vi "NaCTA_configure.vi"() -> ()   [LabVIEW 2016]
uses:
  Instrument drivers/Arduino/ctls_and_globals/Arduino tx msg cluster.ctl
panel:
  in  "Enable USB stream":bool
  in  "n":dbl=0.5
  in  "T0 offset (deg C)":dbl
  in  "P_atmos offset (Pa)":dbl
  in  "Port":refnum<visa-resource-name>
  in  "Get / Set":u8(ring) items=["Get", "Set"]
  in  "Apply temperature corrections":bool=TRUE
  in  "B":dbl=1.0
  in  "A":dbl
  out "Read-back":string
  out "Status comment":string
  in  "Address":u8=1
  # "Use this vi to configure the NaCTA 'hot-thermistor' node\nThese settings are retained in EEPROM and recalled on power-up."
  # "PN 03/02/2017"
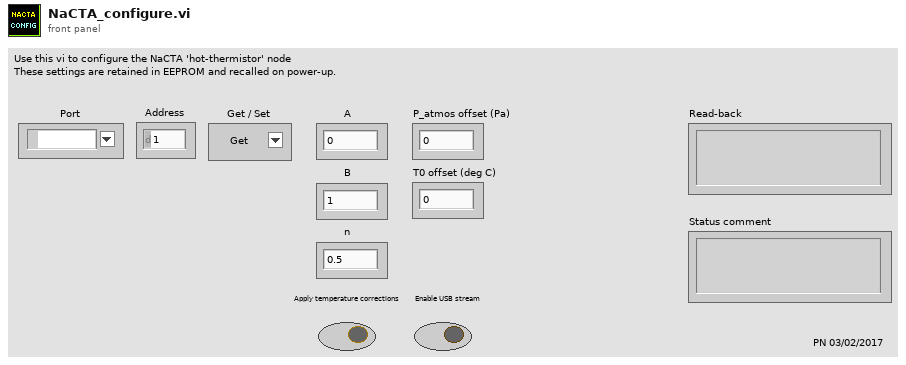
[diagram p1: front panel]
types:
  T1 = typedef "Arduino tx msg cluster.ctl" = cluster{"dest":u8, "A/D/C/I":string, "R/W":string, "chan":u8, "val (float)":sgl}
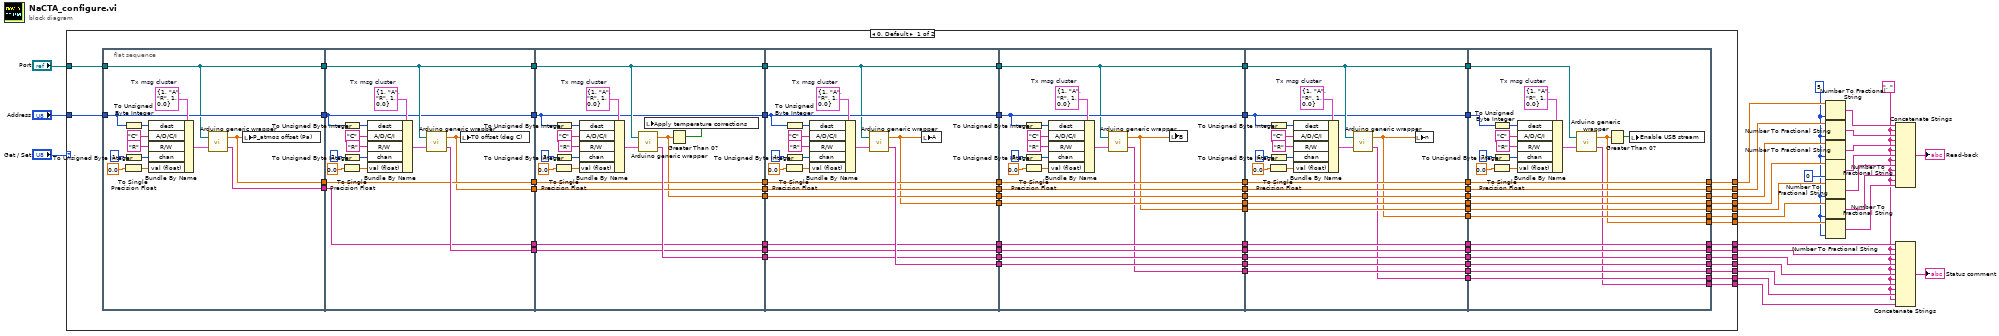
[diagram p0: block diagram]
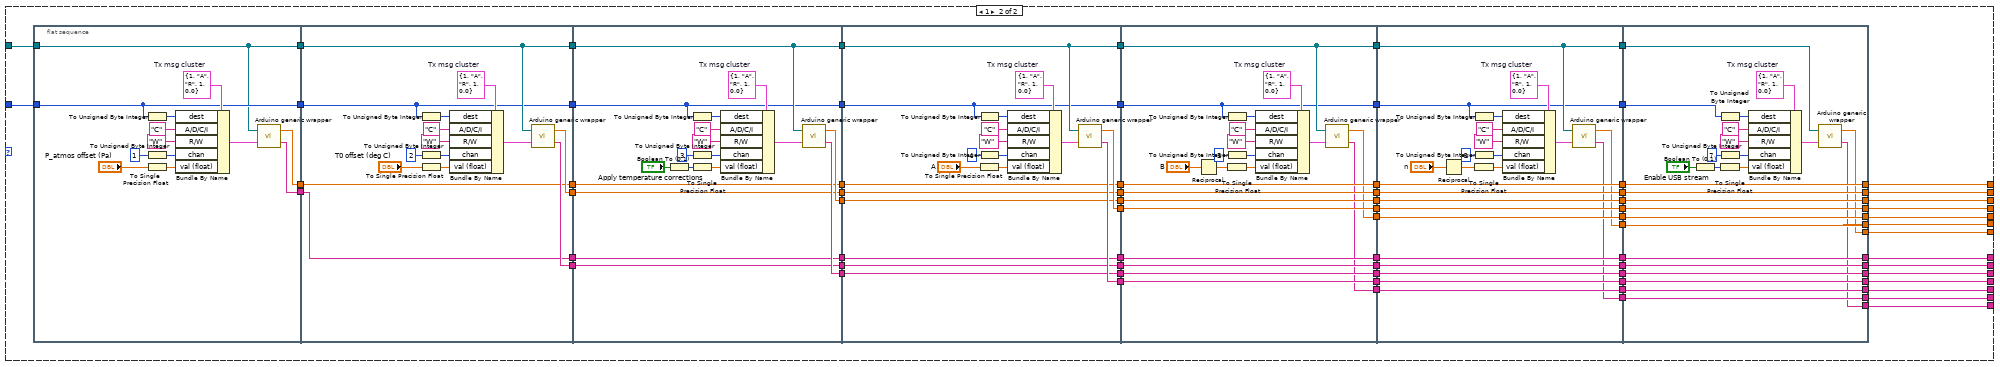
[diagram p2: hidden frame]
diagram:
  w2 = i16 5 ("precision (6)")
  w1 = ", "
  n1 = case shown="0, Default" "Get / Set" {
    tunnel: "Address" -> [w80 w286]
    tunnel: [w72 w285] -> w24
    tunnel: [w76 w284] -> w23
    tunnel: [w77 w283] -> w21
    tunnel: [w73 w282] -> w20
    tunnel: [w74 w281] -> w19
    tunnel: [w75 w280] -> w18
    tunnel: [w78 w279] -> w17
    tunnel: [w79 w278] -> w16
    tunnel: "Port" -> [w81 w277]
    tunnel: [w39 w266] -> w8
    tunnel: [w33 w252] -> w7
    tunnel: [w30 w236] -> w6
    tunnel: [w37 w265] -> w5
    tunnel: [w34 w251] -> w4
    tunnel: [w31 w235] -> w3
    frame 0, Default {
      n2 = flat-sequence {
        tunnel: w80 -> [w104]
        tunnel: w81 -> [w103]
        tunnel: [w103] -> w99
        tunnel: [w104] -> w98
        tunnel: [w100] -> w97
        tunnel: [w102] -> w96
        tunnel: [w119] -> w95
        tunnel: [w118] -> w94
        tunnel: [w117] -> w93
        tunnel: [w113] -> w92
        tunnel: w99 -> [w119]
        tunnel: w98 -> [w118]
        tunnel: w97 -> [w115]
        tunnel: w96 -> [w116]
        tunnel: [w116] -> w91
        tunnel: [w115] -> w90
        tunnel: w95 -> [w137]
        tunnel: [w137] -> w89
        tunnel: w94 -> [w136]
        tunnel: [w136] -> w88
        tunnel: w93 -> [w134]
        tunnel: w92 -> [w132]
        tunnel: [w135] -> w87
        tunnel: [w128] -> w86
        tunnel: [w134] -> w85
        tunnel: [w133] -> w84
        tunnel: w91 -> [w133]
        tunnel: [w132] -> w83
        tunnel: [w131] -> w82
        tunnel: w90 -> [w131]
        tunnel: w89 -> [w147]
        tunnel: w88 -> [w148]
        tunnel: w87 -> [w154]
        tunnel: w86 -> [w155]
        tunnel: w85 -> [w153]
        tunnel: w84 -> [w152]
        tunnel: w83 -> [w151]
        tunnel: w82 -> [w150]
        tunnel: [w156] -> w71
        tunnel: [w146] -> w70
        tunnel: [w155] -> w69
        tunnel: [w154] -> w68
        tunnel: [w153] -> w67
        tunnel: [w152] -> w66
        tunnel: [w151] -> w65
        tunnel: [w150] -> w64
        tunnel: [w148] -> w47
        tunnel: [w147] -> w46
        tunnel: w71 -> [w185]
        tunnel: w70 -> [w184]
        tunnel: w69 -> [w183]
        tunnel: w68 -> [w182]
        tunnel: w67 -> [w181]
        tunnel: w66 -> [w180]
        tunnel: w65 -> [w179]
        tunnel: w64 -> [w178]
        tunnel: [w185] -> w63
        tunnel: [w184] -> w62
        tunnel: [w183] -> w61
        tunnel: [w182] -> w60
        tunnel: [w181] -> w59
        tunnel: [w180] -> w58
        tunnel: [w179] -> w57
        tunnel: [w178] -> w56
        tunnel: w47 -> [w168]
        tunnel: w46 -> [w167]
        tunnel: [w168] -> w45
        tunnel: [w167] -> w44
        tunnel: [w166] -> w41
        tunnel: [w165] -> w40
        tunnel: w63 -> [w208]
        tunnel: w62 -> [w207]
        tunnel: w61 -> [w206]
        tunnel: w60 -> [w205]
        tunnel: w59 -> [w204]
        tunnel: w58 -> [w203]
        tunnel: w57 -> [w202]
        tunnel: w56 -> [w201]
        tunnel: [w208] -> w55
        tunnel: [w207] -> w54
        tunnel: [w206] -> w53
        tunnel: [w205] -> w52
        tunnel: [w204] -> w51
        tunnel: [w203] -> w50
        tunnel: [w202] -> w49
        tunnel: [w201] -> w48
        tunnel: w45 -> [w188]
        tunnel: w44 -> [w189]
        tunnel: [w188] -> w43
        tunnel: [w189] -> w42
        tunnel: w41 -> [w200]
        tunnel: w40 -> [w199]
        tunnel: [w200] -> w38
        tunnel: [w199] -> w36
        tunnel: [w187] -> w35
        tunnel: [w186] -> w32
        tunnel: w55 -> [w234]
        tunnel: w54 -> [w233]
        tunnel: w53 -> [w232]
        tunnel: w52 -> [w231]
        tunnel: w51 -> [w230]
        tunnel: w50 -> [w229]
        tunnel: w49 -> [w228]
        tunnel: w48 -> [w227]
        tunnel: w43 -> [w212]
        tunnel: w42 -> [w211]
        tunnel: w38 -> [w226]
        tunnel: w36 -> [w225]
        tunnel: w35 -> [w224]
        tunnel: w32 -> [w223]
        tunnel: [w213] -> w30
        tunnel: [w209] -> w31
        tunnel: [w223] -> w33
        tunnel: [w224] -> w34
        tunnel: [w225] -> w37
        tunnel: [w226] -> w39
        tunnel: [w227] -> w79
        tunnel: [w228] -> w78
        tunnel: [w229] -> w75
        tunnel: [w230] -> w74
        tunnel: [w231] -> w73
        tunnel: [w232] -> w77
        tunnel: [w233] -> w76
        tunnel: [w234] -> w72
        frame #0 {
          w112 = T1 {"dest"=1, "A/D/C/I"="A", "R/W"="R", "chan"=1, "val (float)"=0.0}  # Tx msg cluster
          n3 = To Unsigned Byte Integer(number=w104) -> (unsigned 8bit integer=w110:u8)
          n4 = To Unsigned Byte Integer(number=u8 1) -> (unsigned 8bit integer=w111:u8)
          n5 = To Single Precision Float(number=0.0) -> (single precision float=w108:sgl)
          n6 = Bundle By Name(cluster=w112, "dest"=w110, "A/D/C/I"="C" ("A/D"), "R/W"="R", "chan"=w111, "val (float)"=w108) -> (w109:T1)
          n7 = call "Arduino generic wrapper.vi"("Tx msg cluster"=w109, "Port name"=w103) -> ("Scan comment"=w102:string, "Output"=w100:dbl)
          n8 = local write "P_atmos offset (Pa)"(w100) -> ()
        }
        frame #1 {
          w120 = T1 {"dest"=1, "A/D/C/I"="A", "R/W"="R", "chan"=1, "val (float)"=0.0}  # Tx msg cluster
          n9 = To Unsigned Byte Integer(number=w118) -> (unsigned 8bit integer=w122:u8)
          n10 = To Unsigned Byte Integer(number=u8 2) -> (unsigned 8bit integer=w121:u8)
          n11 = To Single Precision Float(number=0.0) -> (single precision float=w124:sgl)
          n12 = Bundle By Name(cluster=w120, "dest"=w122, "A/D/C/I"="C" ("A/D"), "R/W"="R", "chan"=w121, "val (float)"=w124) -> (w123:T1)
          n13 = call "Arduino generic wrapper.vi"("Tx msg cluster"=w123, "Port name"=w119) -> ("Scan comment"=w117:string, "Output"=w113:dbl)
          n14 = local write "T0 offset (deg C)"(w113) -> ()
        }
        frame #2 {
          w145 = T1 {"dest"=1, "A/D/C/I"="A", "R/W"="R", "chan"=1, "val (float)"=0.0}  # Tx msg cluster
          n15 = To Unsigned Byte Integer(number=w136) -> (unsigned 8bit integer=w143:u8)
          n16 = To Unsigned Byte Integer(number=u8 3) -> (unsigned 8bit integer=w144:u8)
          n17 = To Single Precision Float(number=0.0) -> (single precision float=w141:sgl)
          n18 = Bundle By Name(cluster=w145, "dest"=w143, "A/D/C/I"="C" ("A/D"), "R/W"="R", "chan"=w144, "val (float)"=w141) -> (w142:T1)
          n19 = call "Arduino generic wrapper.vi"("Tx msg cluster"=w142, "Port name"=w137) -> ("Scan comment"=w135:string, "Output"=w128:dbl)
          n20 = Greater Than 0?(x=w128) -> (x > 0?=w129:bool)
          n21 = local write "Apply temperature corrections"(w129) -> ()
        }
        frame #3 {
          w163 = T1 {"dest"=1, "A/D/C/I"="A", "R/W"="R", "chan"=1, "val (float)"=0.0}  # Tx msg cluster
          n22 = To Unsigned Byte Integer(number=w148) -> (unsigned 8bit integer=w157:u8)
          n23 = To Unsigned Byte Integer(number=u8 4) -> (unsigned 8bit integer=w158:u8)
          n24 = To Single Precision Float(number=0.0) -> (single precision float=w160:sgl)
          n25 = Bundle By Name(cluster=w163, "dest"=w157, "A/D/C/I"="C" ("A/D"), "R/W"="R", "chan"=w158, "val (float)"=w160) -> (w159:T1)
          n26 = call "Arduino generic wrapper.vi"("Tx msg cluster"=w159, "Port name"=w147) -> ("Scan comment"=w156:string, "Output"=w146:dbl)
          n27 = local write "A"(w146) -> ()
        }
        frame #4 {
          w170 = T1 {"dest"=1, "A/D/C/I"="A", "R/W"="R", "chan"=1, "val (float)"=0.0}  # Tx msg cluster
          n28 = To Unsigned Byte Integer(number=w168) -> (unsigned 8bit integer=w176:u8)
          n29 = To Unsigned Byte Integer(number=u8 5) -> (unsigned 8bit integer=w175:u8)
          n30 = To Single Precision Float(number=0.0) -> (single precision float=w173:sgl)
          n31 = Bundle By Name(cluster=w170, "dest"=w176, "A/D/C/I"="C" ("A/D"), "R/W"="R", "chan"=w175, "val (float)"=w173) -> (w174:T1)
          n32 = call "Arduino generic wrapper.vi"("Tx msg cluster"=w174, "Port name"=w167) -> ("Scan comment"=w166:string, "Output"=w165:dbl)
          n33 = local write "B"(w165) -> ()
        }
        frame #5 {
          w197 = T1 {"dest"=1, "A/D/C/I"="A", "R/W"="R", "chan"=1, "val (float)"=0.0}  # Tx msg cluster
          n34 = To Unsigned Byte Integer(number=w188) -> (unsigned 8bit integer=w191:u8)
          n35 = To Unsigned Byte Integer(number=u8 6) -> (unsigned 8bit integer=w192:u8)
          n36 = To Single Precision Float(number=0.0) -> (single precision float=w194:sgl)
          n37 = Bundle By Name(cluster=w197, "dest"=w191, "A/D/C/I"="C" ("A/D"), "R/W"="R", "chan"=w192, "val (float)"=w194) -> (w193:T1)
          n38 = call "Arduino generic wrapper.vi"("Tx msg cluster"=w193, "Port name"=w189) -> ("Scan comment"=w186:string, "Output"=w187:dbl)
          n39 = local write "n"(w187) -> ()
        }
        frame #6 {
          w215 = T1 {"dest"=1, "A/D/C/I"="A", "R/W"="R", "chan"=1, "val (float)"=0.0}  # Tx msg cluster
          n40 = To Unsigned Byte Integer(number=w212) -> (unsigned 8bit integer=w221:u8)
          n41 = To Unsigned Byte Integer(number=u8 7) -> (unsigned 8bit integer=w220:u8)
          n42 = To Single Precision Float(number=0.0) -> (single precision float=w218:sgl)
          n43 = Bundle By Name(cluster=w215, "dest"=w221, "A/D/C/I"="C" ("A/D"), "R/W"="R", "chan"=w220, "val (float)"=w218) -> (w219:T1)
          n44 = call "Arduino generic wrapper.vi"("Tx msg cluster"=w219, "Port name"=w211) -> ("Scan comment"=w213:string, "Output"=w209:dbl)
          n45 = Greater Than 0?(x=w209) -> (x > 0?=w210:bool)
          n46 = local write "Enable USB stream"(w210) -> ()
        }
      }
    }
    frame 1 {
      n47 = flat-sequence {
        tunnel: w286 -> [w309]
        tunnel: w277 -> [w308]
        tunnel: [w308] -> w304
        tunnel: [w309] -> w303
        tunnel: [w307] -> w302
        tunnel: [w306] -> w301
        tunnel: [w324] -> w300
        tunnel: [w323] -> w299
        tunnel: [w322] -> w298
        tunnel: [w321] -> w297
        tunnel: w304 -> [w324]
        tunnel: w303 -> [w323]
        tunnel: w302 -> [w319]
        tunnel: w301 -> [w320]
        tunnel: [w320] -> w296
        tunnel: [w319] -> w295
        tunnel: w300 -> [w342]
        tunnel: [w342] -> w294
        tunnel: w299 -> [w341]
        tunnel: [w341] -> w293
        tunnel: w298 -> [w338]
        tunnel: w297 -> [w336]
        tunnel: [w340] -> w292
        tunnel: [w339] -> w291
        tunnel: [w338] -> w290
        tunnel: [w337] -> w289
        tunnel: w296 -> [w337]
        tunnel: [w336] -> w288
        tunnel: [w335] -> w287
        tunnel: w295 -> [w335]
        tunnel: w294 -> [w353]
        tunnel: w293 -> [w352]
        tunnel: w292 -> [w358]
        tunnel: w291 -> [w359]
        tunnel: w290 -> [w357]
        tunnel: w289 -> [w356]
        tunnel: w288 -> [w355]
        tunnel: w287 -> [w354]
        tunnel: [w361] -> w276
        tunnel: [w360] -> w275
        tunnel: [w359] -> w274
        tunnel: [w358] -> w273
        tunnel: [w357] -> w272
        tunnel: [w356] -> w271
        tunnel: [w355] -> w270
        tunnel: [w354] -> w269
        tunnel: [w353] -> w268
        tunnel: [w352] -> w267
        tunnel: w276 -> [w391]
        tunnel: w275 -> [w390]
        tunnel: w274 -> [w389]
        tunnel: w273 -> [w388]
        tunnel: w272 -> [w387]
        tunnel: w271 -> [w386]
        tunnel: w270 -> [w385]
        tunnel: w269 -> [w384]
        tunnel: w268 -> [w373]
        tunnel: w267 -> [w372]
        tunnel: [w391] -> w264
        tunnel: [w390] -> w263
        tunnel: [w389] -> w262
        tunnel: [w388] -> w261
        tunnel: [w387] -> w260
        tunnel: [w386] -> w259
        tunnel: [w385] -> w258
        tunnel: [w384] -> w257
        tunnel: [w375] -> w256
        tunnel: [w374] -> w255
        tunnel: [w373] -> w254
        tunnel: [w372] -> w253
        tunnel: w264 -> [w415]
        tunnel: w263 -> [w414]
        tunnel: w262 -> [w413]
        tunnel: w261 -> [w412]
        tunnel: w260 -> [w411]
        tunnel: w259 -> [w410]
        tunnel: w258 -> [w409]
        tunnel: w257 -> [w408]
        tunnel: w256 -> [w407]
        tunnel: w255 -> [w406]
        tunnel: w254 -> [w395]
        tunnel: w253 -> [w394]
        tunnel: [w415] -> w250
        tunnel: [w414] -> w249
        tunnel: [w413] -> w248
        tunnel: [w412] -> w247
        tunnel: [w411] -> w246
        tunnel: [w410] -> w245
        tunnel: [w409] -> w244
        tunnel: [w408] -> w243
        tunnel: [w407] -> w242
        tunnel: [w406] -> w241
        tunnel: [w397] -> w240
        tunnel: [w396] -> w239
        tunnel: [w395] -> w238
        tunnel: [w394] -> w237
        tunnel: w250 -> [w441]
        tunnel: w249 -> [w440]
        tunnel: w248 -> [w439]
        tunnel: w247 -> [w438]
        tunnel: w246 -> [w437]
        tunnel: w245 -> [w436]
        tunnel: w244 -> [w435]
        tunnel: w243 -> [w434]
        tunnel: w242 -> [w433]
        tunnel: w241 -> [w432]
        tunnel: w240 -> [w431]
        tunnel: w239 -> [w430]
        tunnel: w238 -> [w418]
        tunnel: w237 -> [w419]
        tunnel: [w420] -> w235
        tunnel: [w421] -> w236
        tunnel: [w430] -> w251
        tunnel: [w431] -> w252
        tunnel: [w432] -> w265
        tunnel: [w433] -> w266
        tunnel: [w434] -> w278
        tunnel: [w435] -> w279
        tunnel: [w436] -> w280
        tunnel: [w437] -> w281
        tunnel: [w438] -> w282
        tunnel: [w439] -> w283
        tunnel: [w440] -> w284
        tunnel: [w441] -> w285
        frame #0 {
          w317 = T1 {"dest"=1, "A/D/C/I"="A", "R/W"="R", "chan"=1, "val (float)"=0.0}  # Tx msg cluster
          n48 = To Unsigned Byte Integer(number=w309) -> (unsigned 8bit integer=w315:u8)
          n49 = To Unsigned Byte Integer(number=u8 1) -> (unsigned 8bit integer=w316:u8)
          n50 = To Single Precision Float(number="P_atmos offset (Pa)") -> (single precision float=w313:sgl)
          n51 = Bundle By Name(cluster=w317, "dest"=w315, "A/D/C/I"="C" ("A/D"), "R/W"="W", "chan"=w316, "val (float)"=w313) -> (w314:T1)
          n52 = call "Arduino generic wrapper.vi"("Tx msg cluster"=w314, "Port name"=w308) -> ("Scan comment"=w306:string, "Output"=w307:dbl)
        }
        frame #1 {
          w325 = T1 {"dest"=1, "A/D/C/I"="A", "R/W"="R", "chan"=1, "val (float)"=0.0}  # Tx msg cluster
          n53 = To Unsigned Byte Integer(number=w323) -> (unsigned 8bit integer=w327:u8)
          n54 = To Unsigned Byte Integer(number=u8 2) -> (unsigned 8bit integer=w326:u8)
          n55 = To Single Precision Float(number="T0 offset (deg C)") -> (single precision float=w329:sgl)
          n56 = Bundle By Name(cluster=w325, "dest"=w327, "A/D/C/I"="C" ("A/D"), "R/W"="W", "chan"=w326, "val (float)"=w329) -> (w328:T1)
          n57 = call "Arduino generic wrapper.vi"("Tx msg cluster"=w328, "Port name"=w324) -> ("Scan comment"=w322:string, "Output"=w321:dbl)
        }
        frame #2 {
          w350 = T1 {"dest"=1, "A/D/C/I"="A", "R/W"="R", "chan"=1, "val (float)"=0.0}  # Tx msg cluster
          n58 = Boolean To (0,1)(Boolean="Apply temperature corrections") -> (0, 1=w333:i16)
          n59 = To Unsigned Byte Integer(number=w341) -> (unsigned 8bit integer=w348:u8)
          n60 = To Unsigned Byte Integer(number=u8 3) -> (unsigned 8bit integer=w349:u8)
          n61 = To Single Precision Float(number=w333) -> (single precision float=w346:sgl)
          n62 = Bundle By Name(cluster=w350, "dest"=w348, "A/D/C/I"="C" ("A/D"), "R/W"="W", "chan"=w349, "val (float)"=w346) -> (w347:T1)
          n63 = call "Arduino generic wrapper.vi"("Tx msg cluster"=w347, "Port name"=w342) -> ("Scan comment"=w340:string, "Output"=w339:dbl)
        }
        frame #3 {
          w368 = T1 {"dest"=1, "A/D/C/I"="A", "R/W"="R", "chan"=1, "val (float)"=0.0}  # Tx msg cluster
          n64 = To Unsigned Byte Integer(number=w352) -> (unsigned 8bit integer=w362:u8)
          n65 = To Unsigned Byte Integer(number=u8 4) -> (unsigned 8bit integer=w363:u8)
          n66 = To Single Precision Float(number="A") -> (single precision float=w365:sgl)
          n67 = Bundle By Name(cluster=w368, "dest"=w362, "A/D/C/I"="C" ("A/D"), "R/W"="W", "chan"=w363, "val (float)"=w365) -> (w364:T1)
          n68 = call "Arduino generic wrapper.vi"("Tx msg cluster"=w364, "Port name"=w353) -> ("Scan comment"=w361:string, "Output"=w360:dbl)
        }
        frame #4 {
          w377 = T1 {"dest"=1, "A/D/C/I"="A", "R/W"="R", "chan"=1, "val (float)"=0.0}  # Tx msg cluster
          n69 = Reciprocal(x="B") -> (1/x=w371:dbl)
          n70 = To Unsigned Byte Integer(number=w372) -> (unsigned 8bit integer=w383:u8)
          n71 = To Unsigned Byte Integer(number=u8 5) -> (unsigned 8bit integer=w382:u8)
          n72 = To Single Precision Float(number=w371) -> (single precision float=w380:sgl)
          n73 = Bundle By Name(cluster=w377, "dest"=w383, "A/D/C/I"="C" ("A/D"), "R/W"="W", "chan"=w382, "val (float)"=w380) -> (w381:T1)
          n74 = call "Arduino generic wrapper.vi"("Tx msg cluster"=w381, "Port name"=w373) -> ("Scan comment"=w375:string, "Output"=w374:dbl)
        }
        frame #5 {
          w404 = T1 {"dest"=1, "A/D/C/I"="A", "R/W"="R", "chan"=1, "val (float)"=0.0}  # Tx msg cluster
          n75 = Reciprocal(x="n") -> (1/x=w393:dbl)
          n76 = To Unsigned Byte Integer(number=w394) -> (unsigned 8bit integer=w398:u8)
          n77 = To Unsigned Byte Integer(number=u8 6) -> (unsigned 8bit integer=w399:u8)
          n78 = To Single Precision Float(number=w393) -> (single precision float=w401:sgl)
          n79 = Bundle By Name(cluster=w404, "dest"=w398, "A/D/C/I"="C" ("A/D"), "R/W"="W", "chan"=w399, "val (float)"=w401) -> (w400:T1)
          n80 = call "Arduino generic wrapper.vi"("Tx msg cluster"=w400, "Port name"=w395) -> ("Scan comment"=w397:string, "Output"=w396:dbl)
        }
        frame #6 {
          w423 = T1 {"dest"=1, "A/D/C/I"="A", "R/W"="R", "chan"=1, "val (float)"=0.0}  # Tx msg cluster
          n81 = Boolean To (0,1)(Boolean="Enable USB stream") -> (0, 1=w417:i16)
          n82 = To Unsigned Byte Integer(number=w419) -> (unsigned 8bit integer=w429:u8)
          n83 = To Unsigned Byte Integer(number=u8 7) -> (unsigned 8bit integer=w428:u8)
          n84 = To Single Precision Float(number=w417) -> (single precision float=w426:sgl)
          n85 = Bundle By Name(cluster=w423, "dest"=w429, "A/D/C/I"="C" ("A/D"), "R/W"="W", "chan"=w428, "val (float)"=w426) -> (w427:T1)
          n86 = call "Arduino generic wrapper.vi"("Tx msg cluster"=w427, "Port name"=w418) -> ("Scan comment"=w421:string, "Output"=w420:dbl)
        }
      }
    }
  }
  n87 = Number To Fractional String(number=w16, precision (6)=w2) -> (F-format string=w28:string)  [unwired: 2 in]
  n88 = Number To Fractional String(number=w17, precision (6)=w2) -> (F-format string=w27:string)  [unwired: 2 in]
  n89 = Number To Fractional String(number=w21, precision (6)=w2) -> (F-format string=w15:string)  [unwired: 2 in]
  n90 = Number To Fractional String(number=w23, precision (6)=i16 0) -> (F-format string=w14:string)  [unwired: 2 in]
  n91 = Number To Fractional String(number=w5, precision (6)=w2) -> (F-format string=w11:string)  [unwired: 2 in]
  n92 = Number To Fractional String(number=w4, precision (6)=w2) -> (F-format string=w10:string)  [unwired: 2 in]
  n93 = Number To Fractional String(number=w3, precision (6)=w2) -> (F-format string=w9:string)  [unwired: 2 in]
  n94 = Concatenate Strings(w28, w1, w27, w1, w15, w1, w14, w1, w11, w1, w10, w1, w9) -> (→"Read-back":string)
  n95 = Concatenate Strings(w18, w1, w19, w1, w20, w1, w24, w1, w8, w1, w7, w1, w6) -> (→"Status comment":string)
